vi "host.vi"() -> ()   [LabVIEW 2020]
uses:
  <vilib>/rvi/interface/RandomDataEmulation/nirviRandomDataOpen.vi
  <vilib>/rvi/interface/common/niFpgaCacheSessionInfoDynamic.vi
  <vilib>/Utility/error.llb/Error Cluster From Error Code.vi
  <vilib>/rvi/errors/niLvFpgaAdjustHostInterfaceError.vi
  <vilib>/FPGAPlugInAG/Dynamic/niLvFpga_Close_Dynamic.vi
  <vilib>/rvi/interface/nirviOpenFPGA/nirviOpenFPGA.xnode
  awgn.vi
  <vilib>/rvi/interface/nirviReadWriteControl/nirviReadWriteControl.xnode
  <vilib>/rvi/interface/nirviMethod/nirviMethod.xnode
  <vilib>/rvi/interface/nirviCloseFPGA/nirviCloseFPGA.xnode
  <vilib>/FPGAPlugInAG/Dynamic/niLvFpga_ReadFifo_Dynamic.vi
  <vilib>/rvi/errors/niLvFpgaMergeErrorWithErrorCode.vi
  NiFpgaLv.dll
  <vilib>/rvi/interface/Simulation/niFpgaSimulationCallBeginRW.vi
panel:
  in  "std":fxp<+,8,8>=1.0
  in  "y":u32=32
  out "?":cluster{i32[], dbl[]}(graph)
  out "?":cluster{dbl[], dbl[]}[](graph)
  out "?":cluster{dbl[], dbl[]}[](graph)
  out "?":cluster{i32[], dbl[]}(graph)
  out "?":cluster{i32[], dbl[]}[](graph)
  out "?":cluster{i32[], dbl[]}[](graph)
  out "?":cluster{i32[], dbl[]}(graph)
  in  "?":bool
  in  "batch size":u32=100
  # "Z0 and Z1 Time domain"
  # "Z0+Z1*i spectrum"
  # "Z0 and Z1 CDF"
  # "Z0+Z1*i transformed spectrum"
  # "U1 and U2 CDF"
  # "U1 and U2 Time domain"
  # "U1+U2*i spectrum"
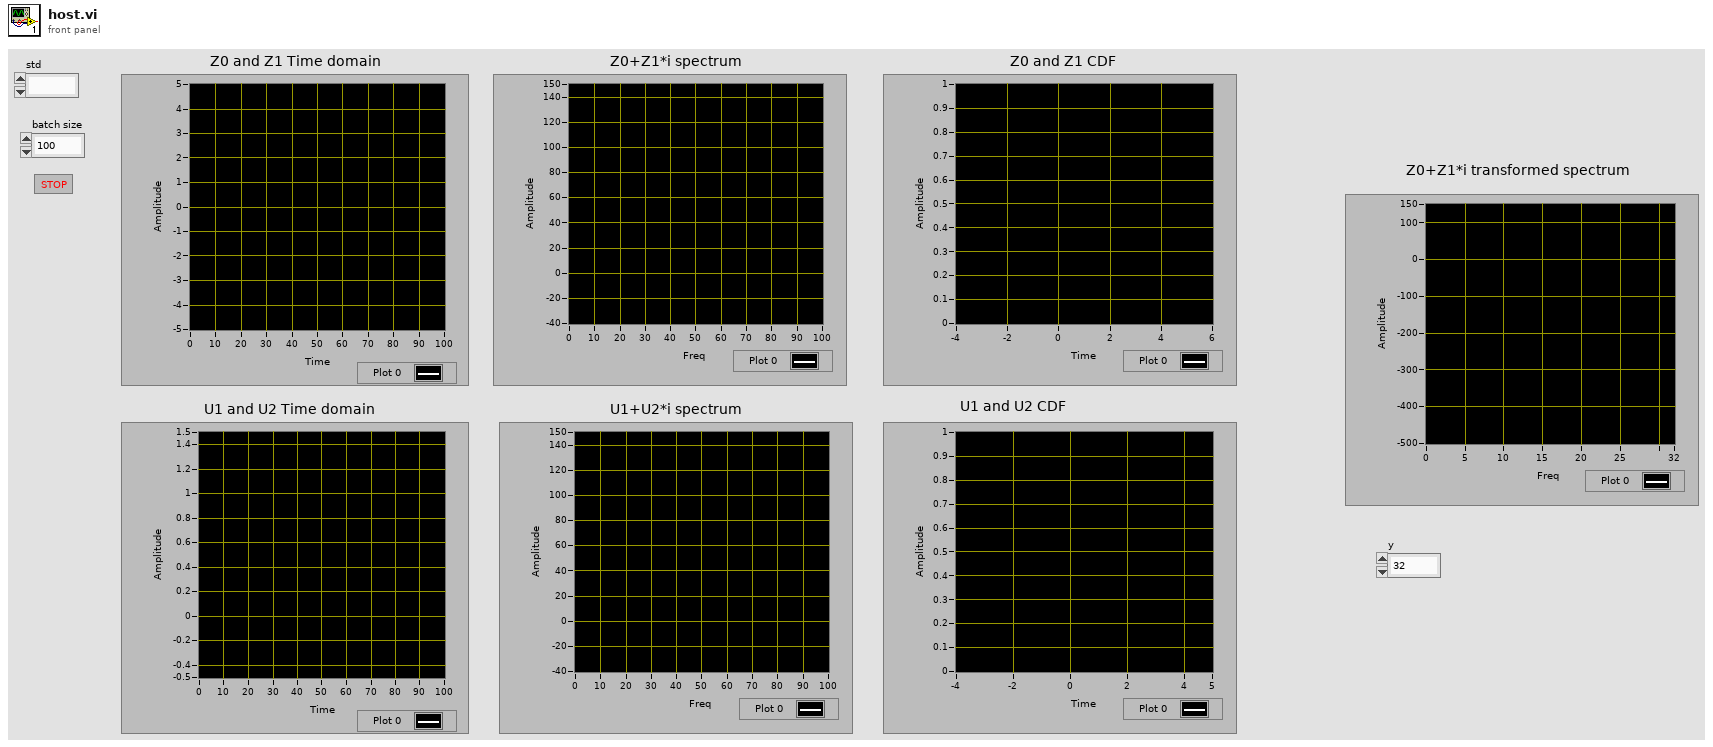
[diagram p1: front panel]
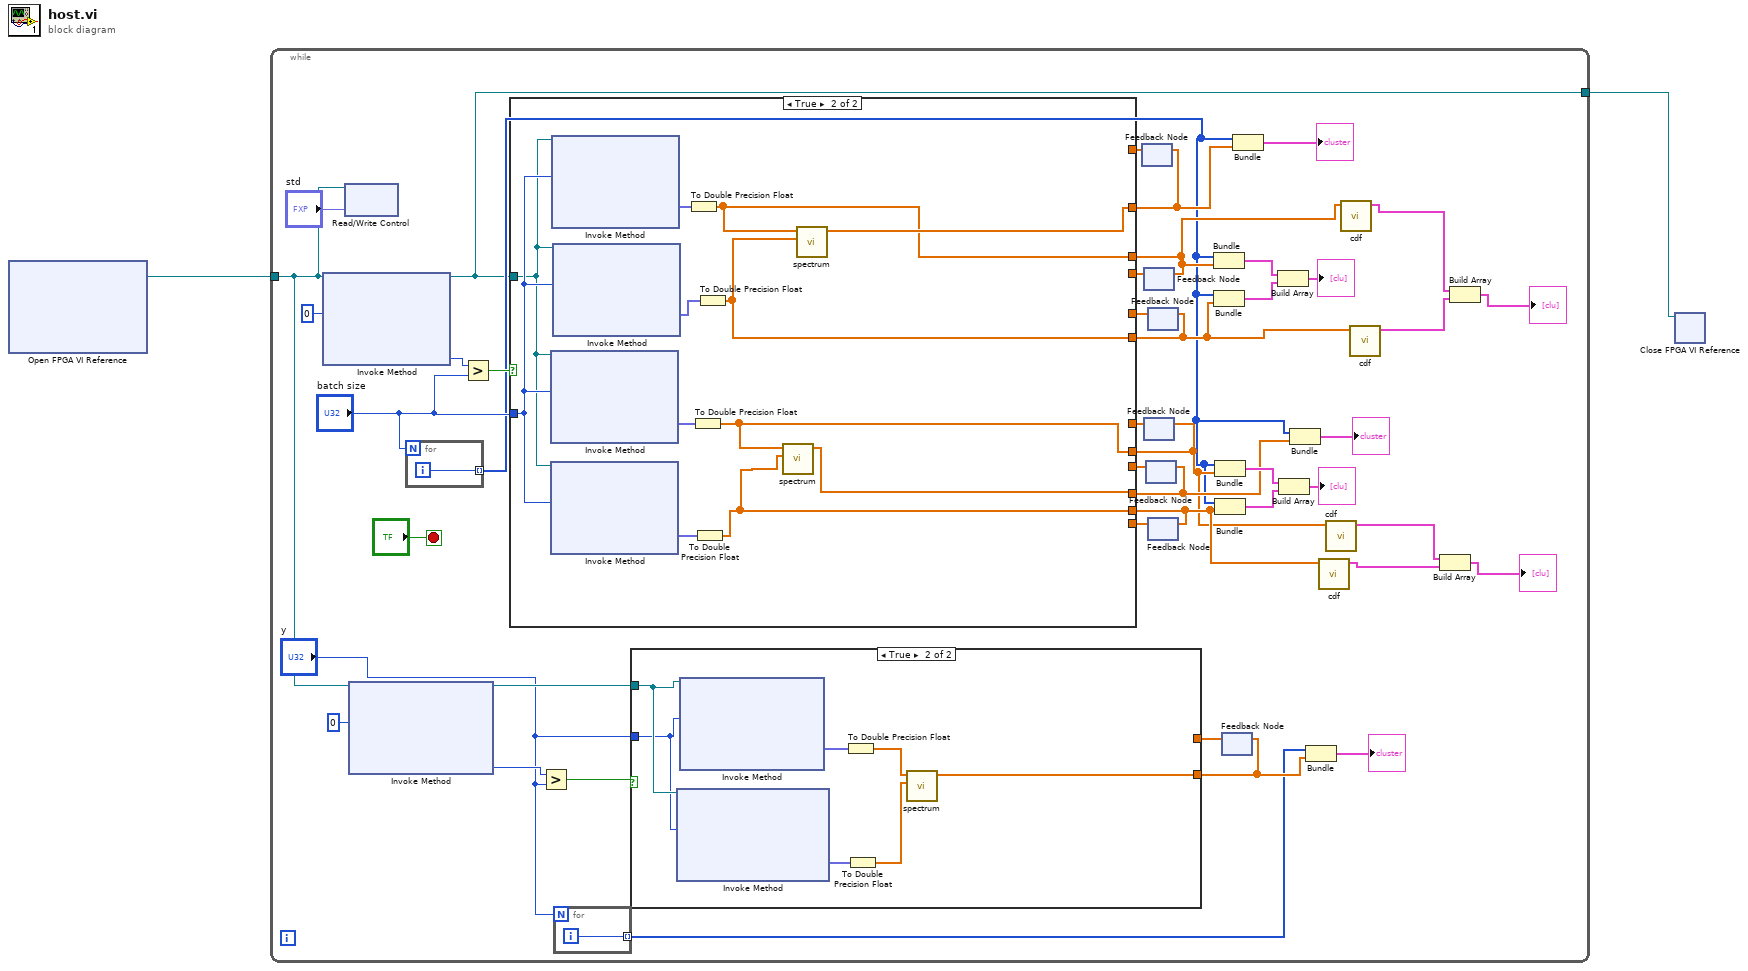
[diagram p0: block diagram]
diagram:
  n1 = xnode "Open FPGA VI Reference"() -> ("FPGA VI Reference Out"=w2:refnum<k20>)  [unwired: 2 in, 1 out]
  n2 = while {
    tunnel: w2 -> [w5]
    tunnel: [w3] -> w1
    stop <- "?" stop-if-true
    n3 = xnode "Invoke Method"("FPGA VI Reference In"=w5, "Number of Elements"=u32 0) -> ("FPGA VI Reference Out"=w3:refnum<k20>, "Elements Remaining"=w45:u32)  [unwired: 2 in, 2 out]
    n4 = xnode "Read/Write Control"("FPGA VI Reference In"=w5, "std"="std") -> ()  [unwired: 1 in, 2 out]
    n5 = xnode "Invoke Method"("FPGA VI Reference In"=w5, "Number of Elements"=u32 0) -> ("FPGA VI Reference Out"=w13:refnum<k20>, "Elements Remaining"=w15:u32)  [unwired: 2 in, 2 out]
    n6 = for {
      N: "batch size" -> [_]
      tunnel: [w56] -> w7 mode=indexing
      i -> [w56]
    }
    n7 = Greater?(x=w45, y="batch size") -> (0:w44:bool)
    n8 = Greater?(x=w15, y="y") -> (0:w14:bool)
    n9 = for {
      N: "y" -> [_]
      tunnel: [w47] -> w6 mode=indexing
      i -> [w47]
    }
    n10 = feedback #1() -> (w42:dbl[])  [unwired: 1 in]
    n11 = feedback #2() -> (w39:dbl[])  [unwired: 1 in]
    n12 = feedback #3() -> (w31:dbl[])  [unwired: 1 in]
    n13 = feedback #4() -> (w28:dbl[])  [unwired: 1 in]
    n14 = feedback #5() -> (w38:dbl[])  [unwired: 1 in]
    n15 = feedback #6() -> (w30:dbl[])  [unwired: 1 in]
    n16 = case shown="True" w44 {
      tunnel: "batch size" -> [_ w74]
      tunnel: w3 -> [_ w73]
      tunnel: [w62 w67] -> w40
      tunnel: w42 -> [w62 _]
      tunnel: [w61 w66] -> w21
      tunnel: [w60 w70] -> w26
      tunnel: w39 -> [w61 _]
      tunnel: w38 -> [w60 _]
      tunnel: [w58 w64] -> w20
      tunnel: [w59 w65] -> w19
      tunnel: w31 -> [w59 _]
      tunnel: w30 -> [w58 _]
      tunnel: [w57 w63] -> w29
      tunnel: w28 -> [w57 _]
      frame False {
      }
      frame True {
        n17 = xnode "Invoke Method"("FPGA VI Reference In"=w73, "Number of Elements"=w74) -> ("Data"=w68:fxp<+,8,0>[])  [unwired: 2 in, 3 out]
        n18 = xnode "Invoke Method"("FPGA VI Reference In"=w73, "Number of Elements"=w74) -> ("Data"=w69:fxp<+,8,0>[])  [unwired: 2 in, 3 out]
        n19 = xnode "Invoke Method"("FPGA VI Reference In"=w73, "Number of Elements"=w74) -> ("Data"=w72:fxp<+/-,44,12>[])  [unwired: 2 in, 3 out]
        n20 = xnode "Invoke Method"("FPGA VI Reference In"=w73, "Number of Elements"=w74) -> ("Data"=w71:fxp<+/-,44,12>[])  [unwired: 2 in, 3 out]
        n21 = To Double Precision Float(number=w72) -> (double precision float=w66:dbl[])
        n22 = To Double Precision Float(number=w68) -> (double precision float=w65:dbl[])
        n23 = To Double Precision Float(number=w69) -> (double precision float=w64:dbl[])
        n24 = To Double Precision Float(number=w71) -> (double precision float=w70:dbl[])
        n25 = call "spectrum.vi"("im"=w64, "re"=w65) -> ("spectrum"=w63:dbl[])  [unwired: 9 in]
        n26 = call "spectrum.vi"("im"=w70, "re"=w66) -> ("spectrum"=w67:dbl[])  [unwired: 9 in]
      }
    }
    n27 = feedback-in #1(w40) -> ()
    n28 = feedback-in #2(w21) -> ()
    n29 = feedback-in #3(w19) -> ()
    n30 = feedback-in #4(w29) -> ()
    n31 = feedback-in #5(w26) -> ()
    n32 = feedback-in #6(w20) -> ()
    n33 = Bundle(w7, w21) -> (w37:cluster{i32[], dbl[]})  [unwired: 1 in]
    n34 = Bundle(w7, w26) -> (w36:cluster{i32[], dbl[]})  [unwired: 1 in]
    n35 = Bundle(w7, w19) -> (w34:cluster{i32[], dbl[]})  [unwired: 1 in]
    n36 = Bundle(w7, w20) -> (w33:cluster{i32[], dbl[]})  [unwired: 1 in]
    n37 = feedback #7() -> (w11:dbl[])  [unwired: 1 in]
    n38 = case shown="True" w14 {
      tunnel: w13 -> [_ w55]
      tunnel: "y" -> [_ w54]
      tunnel: [w48 w49] -> w9
      tunnel: w11 -> [w48 _]
      frame False {
      }
      frame True {
        n39 = xnode "Invoke Method"("FPGA VI Reference In"=w55, "Number of Elements"=w54) -> ("Data"=w52:fxp<+/-,28,17>[])  [unwired: 2 in, 3 out]
        n40 = xnode "Invoke Method"("FPGA VI Reference In"=w55, "Number of Elements"=w54) -> ("Data"=w53:fxp<+/-,28,17>[])  [unwired: 2 in, 3 out]
        n41 = To Double Precision Float(number=w53) -> (double precision float=w51:dbl[])
        n42 = To Double Precision Float(number=w52) -> (double precision float=w50:dbl[])
        n43 = call "spectrum.vi"("im"=w50, "re"=w51) -> ("spectrum"=w49:dbl[])  [unwired: 9 in]
      }
    }
    n44 = feedback-in #7(w9) -> ()
    n45 = Bundle(w7, "spectrum"=w40) -> (→"?":cluster{i32[], "spectrum":dbl[]})  [unwired: 1 in]
    n46 = Build Array(w37, w36) -> (→"?":cluster{i32[], dbl[]}[])
    n47 = Build Array(w34, w33) -> (→"?":cluster{i32[], dbl[]}[])
    n48 = Bundle(w7, "spectrum"=w29) -> (→"?":cluster{i32[], "spectrum":dbl[]})  [unwired: 1 in]
    n49 = Bundle(w6, "spectrum"=w9) -> (→"?":cluster{i32[], "spectrum":dbl[]})  [unwired: 1 in]
    n50 = call "cdf.vi"("Array"=w20) -> ("Cluster"=w17:cluster{dbl[], dbl[]})  [unwired: 10 in]
    n51 = call "cdf.vi"("Array"=w19) -> ("Cluster"=w18:cluster{dbl[], dbl[]})  [unwired: 10 in]
    n52 = call "cdf.vi"("Array"=w21) -> ("Cluster"=w22:cluster{dbl[], dbl[]})  [unwired: 10 in]
    n53 = call "cdf.vi"("Array"=w26) -> ("Cluster"=w25:cluster{dbl[], dbl[]})  [unwired: 10 in]
    n54 = Build Array(w18, w17) -> (→"?":cluster{dbl[], dbl[]}[])
    n55 = Build Array(w22, w25) -> (→"?":cluster{dbl[], dbl[]}[])
  }
  n56 = xnode "Close FPGA VI Reference"("FPGA VI Reference In"=w1) -> ()  [unwired: 1 in, 1 out]
